vi "user input.vi"(8 "error in":errorcluster, 11 "FPGA Interface":T1) -> (0 "error out":errorcluster, 3 "Inputs from system":T2 {"AILimitLow" format="%.0x"; "AILimitHigh" format="%.0x"})   [LabVIEW 2015, in "GPIC ScaleAndLimit runtime.lvclass"]
uses:
  GPIC ScaleAndLimit runtime.lvclass
  input user data.ctl
  Interface/FPGAInterface.ctl
  <vilib>/Utility/error.llb/Error Cluster From Error Code.vi
  <vilib>/rvi/errors/niLvFpgaAdjustHostInterfaceError.vi
  <vilib>/rvi/interface/nirviReadWriteControl/nirviReadWriteControl.xnode
  Interface/ScaleAndLimitInterface.lvlib
  NiFpgaLv.dll
  <vilib>/rvi/interface/Simulation/niFpgaSimulationCallBeginRW.vi
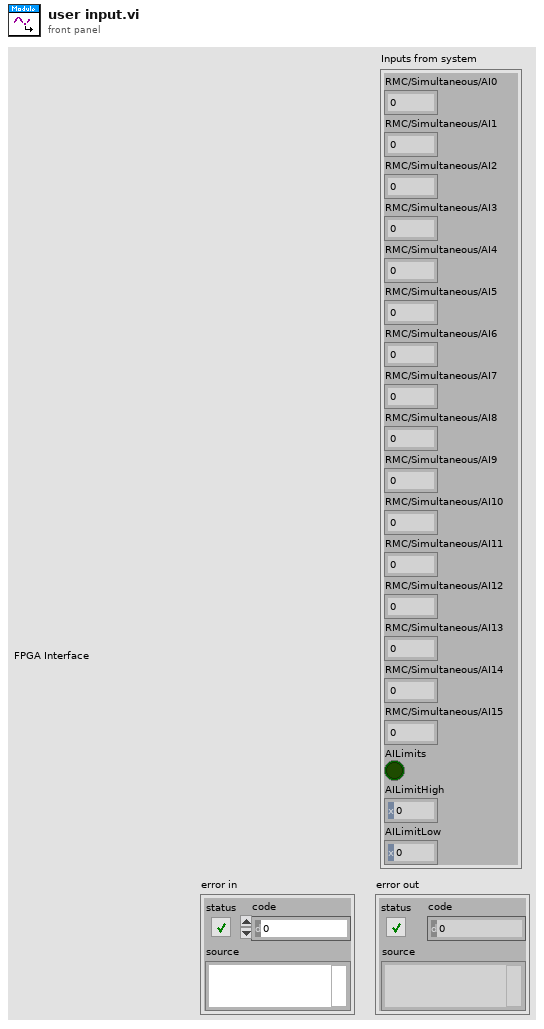
[diagram p1: front panel]
types:
  T1 = typedef "ScaleAndLimitInterface.lvlib/FPGAInterface.ctl" = refnum<k20>
  T2 = typedef "GPIC ScaleAndLimit runtime.lvclass/input user data.ctl" = cluster{"RMC/Simultaneous/AI0":sgl, "RMC/Simultaneous/AI1":sgl, "RMC/Simultaneous/AI2":sgl, "RMC/Simultaneous/AI3":sgl, "RMC/Simultaneous/AI4":sgl, "RMC/Simultaneous/AI5":sgl, "RMC/Simultaneous/AI6":sgl, "RMC/Simultaneous/AI7":sgl, "RMC/Simultaneous/AI8":sgl, "RMC/Simultaneous/AI9":sgl, "RMC/Simultaneous/AI10":sgl, "RMC/Simultaneous/AI11":sgl, "RMC/Simultaneous/AI12":sgl, "RMC/Simultaneous/AI13":sgl, "RMC/Simultaneous/AI14":sgl, "RMC/Simultaneous/AI15":sgl, "AILimits":bool, "AILimitHigh":u16, "AILimitLow":u16}
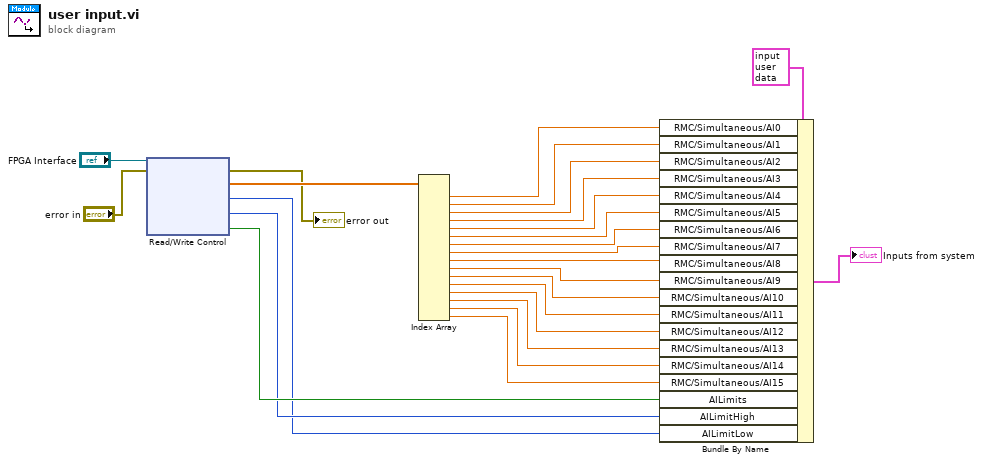
[diagram p0: block diagram]
diagram:
  n1 = xnode "Read/Write Control"("FPGA VI Reference In"="FPGA Interface", "error in"="error in") -> ("error out"=→"error out":errorcluster, "ScaledAI"=w23:sgl[], "AILimitLow"=w1:u16, "AILimitHigh"=w2:u16, "AILimits"=w3:bool)  [unwired: 1 out]
  n2 = Index Array(array=w23) -> (element #1=w20:sgl, element #2=w19:sgl, element #3=w18:sgl, element #4=w16:sgl, element #5=w15:sgl, element #6=w14:sgl, element #7=w13:sgl, element #8=w12:sgl, element #9=w11:sgl, element #10=w10:sgl, element #11=w9:sgl, element #12=w8:sgl, element #13=w7:sgl, element #14=w6:sgl, element #15=w5:sgl, element #16=w4:sgl)  [unwired: 16 in]
  n3 = Bundle By Name(cluster=T2 {"RMC/Simultaneous/AI0"=0.0, "RMC/Simultaneous/AI1"=0.0, "RMC/Simultaneous/AI2"=0.0, "RMC/Simultaneous/AI3"=0.0, "RMC/Simultaneous/AI4"=0.0, "RMC/Simultaneous/AI5"=0.0, "RMC/Simultaneous/AI6"=0.0, "RMC/Simultaneous/AI7"=0.0, "RMC/Simultaneous/AI8"=0.0, "RMC/Simultaneous/AI9"=0.0, "RMC/Simultaneous/AI10"=0.0, "RMC/Simultaneous/AI11"=0.0, "RMC/Simultaneous/AI12"=0.0, "RMC/Simultaneous/AI13"=0.0, "RMC/Simultaneous/AI14"=0.0, "RMC/Simultaneous/AI15"=0.0, "AILimits"=FALSE, "AILimitHigh"=0, "AILimitLow"=0} ("Inputs from system"), "RMC/Simultaneous/AI0"=w20, "RMC/Simultaneous/AI1"=w19, "RMC/Simultaneous/AI2"=w18, "RMC/Simultaneous/AI3"=w16, "RMC/Simultaneous/AI4"=w15, "RMC/Simultaneous/AI5"=w14, "RMC/Simultaneous/AI6"=w13, "RMC/Simultaneous/AI7"=w12, "RMC/Simultaneous/AI8"=w11, "RMC/Simultaneous/AI9"=w10, "RMC/Simultaneous/AI10"=w9, "RMC/Simultaneous/AI11"=w8, "RMC/Simultaneous/AI12"=w7, "RMC/Simultaneous/AI13"=w6, "RMC/Simultaneous/AI14"=w5, "RMC/Simultaneous/AI15"=w4, "AILimits"=w3, "AILimitHigh"=w2, "AILimitLow"=w1) -> (→"Inputs from system":T2)
